vi "Sequence Experiment.getAll.vi"(8 "error in (no error)":errorcluster, 11 "Sequence Experiment":refnum<class "Sequence Experiment.lvclass">) -> (0 "error out":errorcluster, 2 "getAll":T1, 3 "Sequence Experiment out":refnum<class "Sequence Experiment.lvclass">)   [LabVIEW 2016, in "Sequence Experiment.lvclass"]
uses:
  Sequence Experiment.lvclass
  C:/Program Files (x86)/National Instruments/LabVIEW 2016/user.lib/LevyLab/Levylab Instruments/SMOs/Instrument/Instrument.lvclass
  Typedefs/Sequence Experiment.getAll--Cluster.ctl
  <userlib>/LevyLab/Levylab Instruments/SMOs/Instrument/Instrument.lvclass
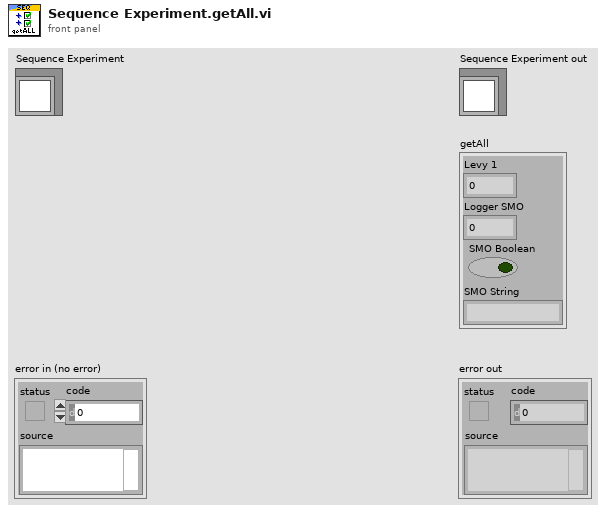
[diagram p1: front panel]
types:
  T1 = typedef "Sequence Experiment.lvclass/Sequence Experiment.getAll--Cluster.ctl" = cluster{"Levy 1":dbl, "Logger SMO":dbl, "SMO Boolean":bool, "SMO String":string}
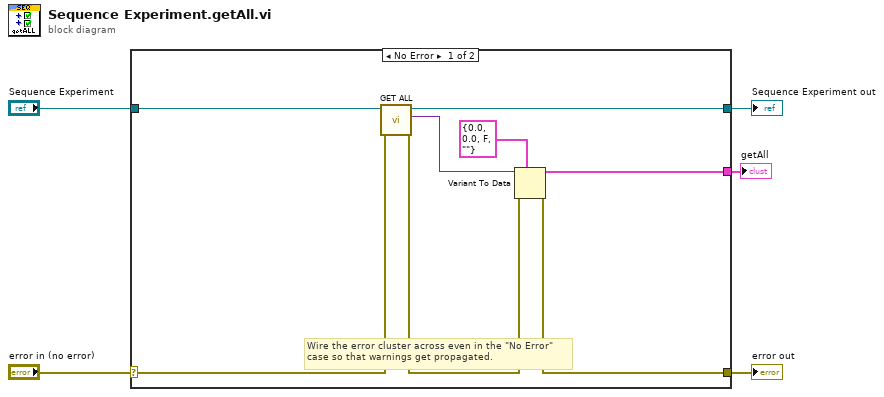
[diagram p0: block diagram]
diagram:
  n1 = case shown="No Error" "error in (no error)" {
    selector: "error in (no error)" -> [w10 w15]
    tunnel: [w8 w15] -> w4
    tunnel: [w11 w14] -> w2
    tunnel: "Sequence Experiment" -> [w12 w14]
    tunnel: [w7 _] -> w1
    frame No Error {
      # "Wire the error cluster across even in the \"No Error\"\ncase so that warnings get propagated."
      n2 = call <userlib>:"GET ALL.vi"("error in (no error)"=w10, "Instrument in"=w12) -> ("error out"=w9:errorcluster, "getAll"=w6:variant, "Instrument out"=w11:refnum<class "Sequence Experiment.lvclass">)  [unwired: 7 in]
      n3 = Variant To Data(error in=w9, type=T1 {"Levy 1"=0.0, "Logger SMO"=0.0, "SMO Boolean"=FALSE, "SMO String"=""} ("getAll"), Variant=w6) -> (data=w7:T1, error out=w8:errorcluster)
    }
    frame Error {
    }
  }
  "error out" <- w4
  "Sequence Experiment out" <- w2
  "getAll" <- w1
